vi "AnimatorCoordinator.vi"(8 "error in (no error)":errorcluster) -> (0 "error out":errorcluster)   [LabVIEW 2019, in "AnimatorXControl.xctl"]
uses:
  AnimatorXControl.xctl
  AnimatorSettings.ctl
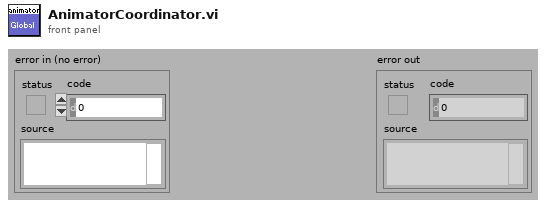
[diagram p1: front panel]
types:
  T1 = typedef "AnimatorXControl.xctl/AnimatorSettings.ctl" = cluster{"Reverse":bool, "FrameRate":dbl, "WorkMode":enum16{"Automatic", "UseValue"}}
  T2 = cluster{"Frame Interval":dbl, "Current Index":u32, "Left Interval":dbl, "Settings":T1}[]
  T3 = cluster{"Picture Ref":refnum<vi>, "PictureArray":picture[]}[]
  T4 = typedef "AnimatorXControl.xctl/QueueElement.ctl" = cluster{"Settings":T1, "Command":T5, "ImageInfo":cluster{"ImageData":picture[], "Pict Refnum":refnum<vi>}, "XRefnum":refnum<vi>}
  T5 = typedef "AnimatorXControl.xctl/AnimatorCommand.ctl" = enum16{"AddAnimator", "RemoveAnimator", "Settings"}
  T6 = cluster{"Frame Interval":dbl, "Current Index":u32, "Left Interval":dbl, "Settings":T1}
  T7 = cluster{"Picture Ref":refnum<vi>, "PictureArray":picture[]}
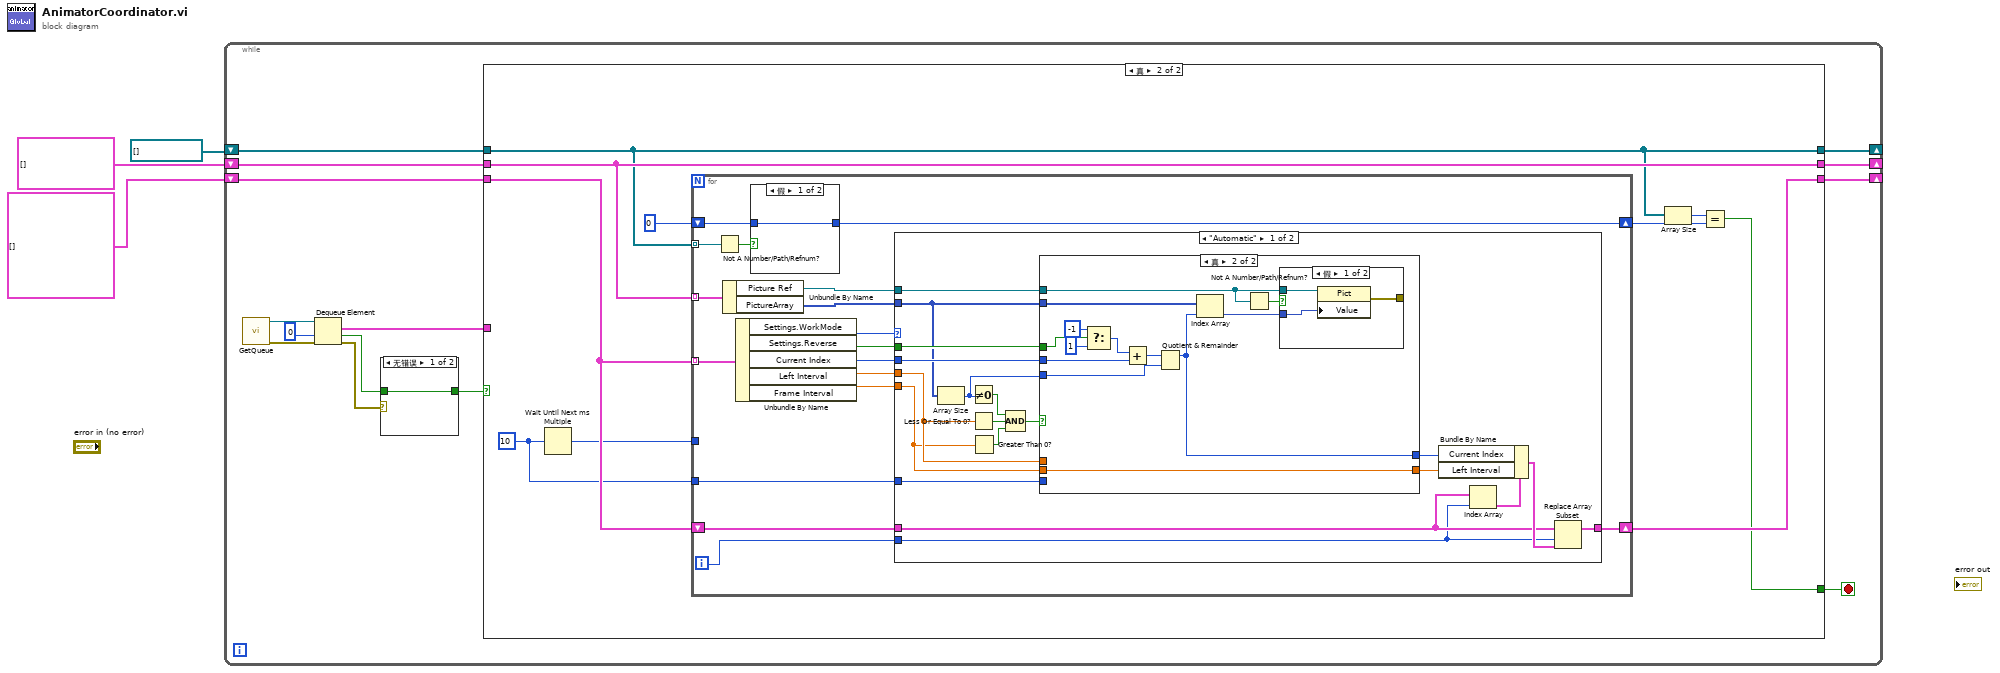
[diagram p0: block diagram]
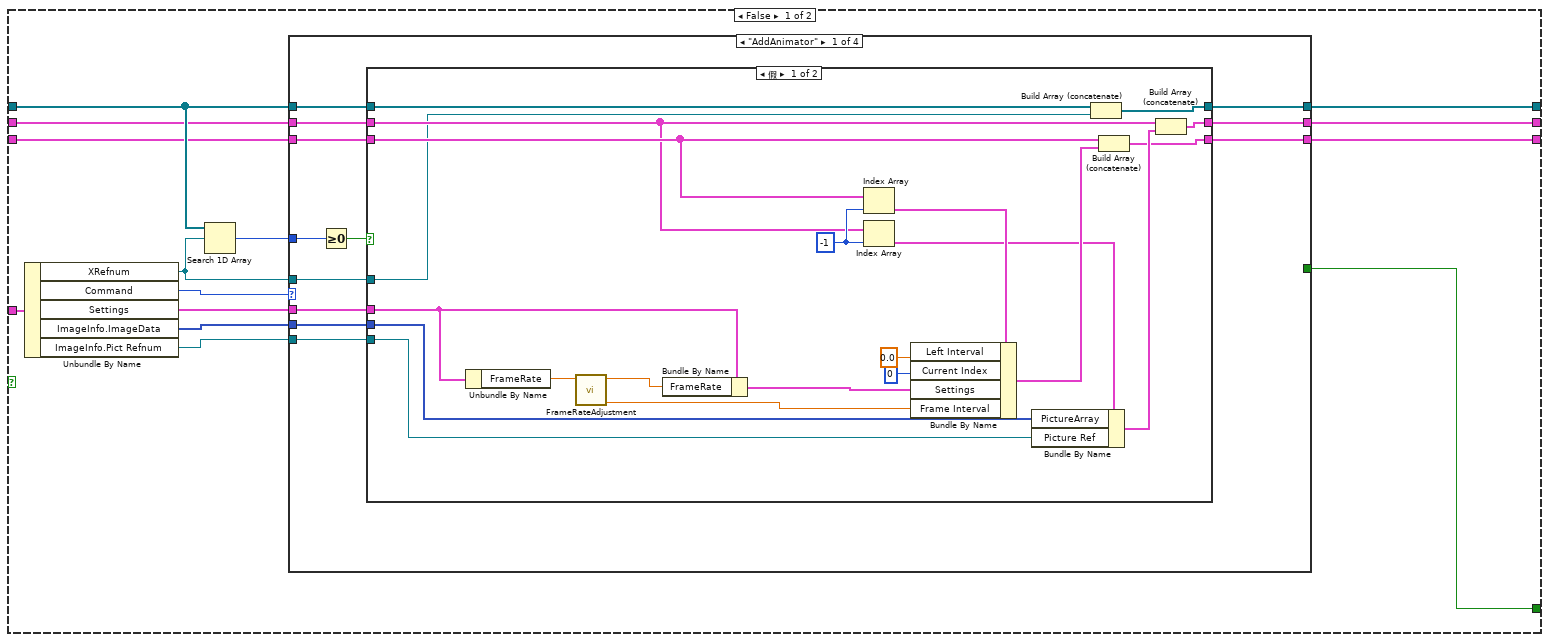
[diagram p2: hidden frame]
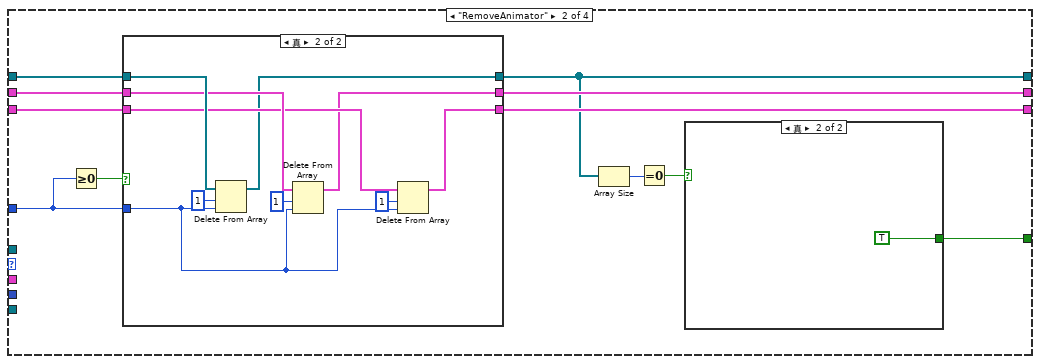
[diagram p4: hidden frame]
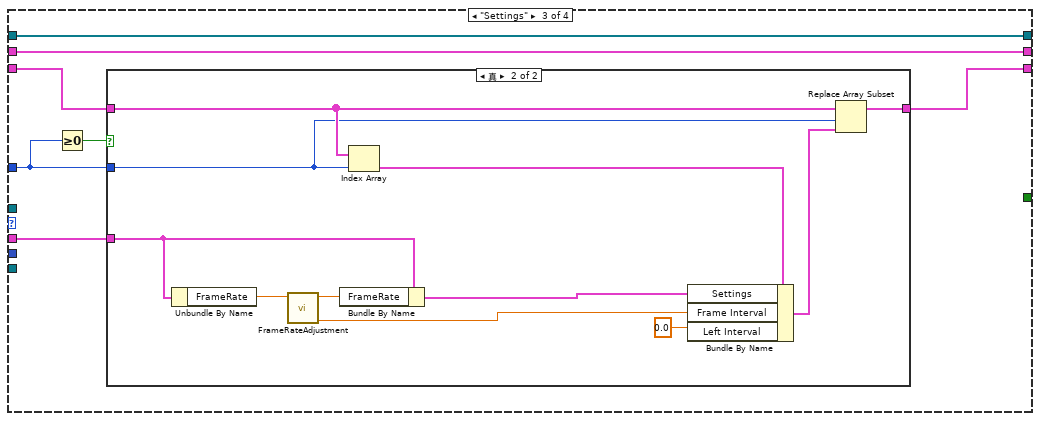
[diagram p7: hidden frame]
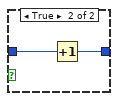
[diagram p10: hidden frame]
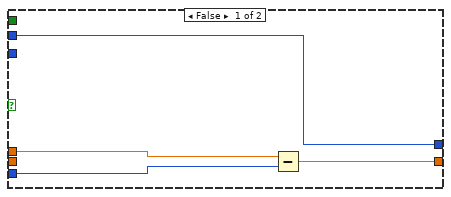
[diagram p11: hidden frame]
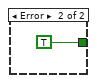
[diagram p14: hidden frame]
diagram:
  n1 = while {
    shift-right: [w15] -> _
    shift-left: refnum<vi>[] [] ("XControlRef Out") -> [w17]
    shift-right: [w13] -> _
    shift-left: T2 [] ("Settings Out") -> [w16]
    shift-right: [w11] -> _
    shift-left: T3 [] ("ImageData Out") -> [w12]
    stop <- w14 stop-if-true
    n2 = call "GetQueue.vi"() -> ("error out"=w8:errorcluster, "queue out"=w10:refnum<queue>)  [unwired: 10 in]
    n3 = Dequeue Element(queue=w10, timeout in ms (-1)=0, error in (no error)=w8) -> (element=w4:T4, timed out?=w6:bool, error out=w7:errorcluster)  [unwired: 1 out]
    n4 = case shown="无错误" w7 {
      tunnel: w6 -> [w185 _]
      tunnel: [w185 TRUE ("timed out?")] -> w5
      frame No Error {
      }
      frame Error {
      }
    }
    n5 = case shown="真" w5 {
      tunnel: w17 -> [w30 w118]
      tunnel: w16 -> [w28 w124]
      tunnel: [w27 w118] -> w15
      tunnel: [w18 w115] -> w14
      tunnel: [w25 w122] -> w13
      tunnel: w12 -> [w29 w123]
      tunnel: [w26 w123] -> w11
      tunnel: w4 -> [w31 _]
      frame False {
        n6 = Unbundle By Name(w31) -> ("XRefnum"=w23:refnum<vi>, "Command"=w24:T5, "Settings"=w20:T1, "ImageInfo.ImageData"=w19:picture[], "ImageInfo.Pict Refnum"=w22:refnum<vi>)
        n7 = Search 1D Array(1D array=w30, element=w23) -> (index of element=w21:i32)  [unwired: 1 in]
        n8 = case shown="\"AddAnimator\"" w24 {
          tunnel: w30 -> [w40 w78 w99 w114]
          tunnel: [w39 w71 w99 w114] -> w27
          tunnel: w29 -> [w41 w77 w97 w113]
          tunnel: w21 -> [w33 w73 w94 _]
          tunnel: [w38 w75 w97 w113] -> w26
          tunnel: w22 -> [w34 _ _ _]
          tunnel: w20 -> [w36 _ w98 _]
          tunnel: w19 -> [w35 _ _ _]
          tunnel: w28 -> [w42 w76 w96 w112]
          tunnel: [w43 w74 w95 w112] -> w25
          tunnel: w23 -> [w37 _ _ _]
          tunnel: [_ w68 _ _] -> w18
          frame "AddAnimator" {
            n9 = Greater Or Equal To 0?(x=w33) -> (x >= 0?=w32:bool)
            n10 = case shown="假" w32 {
              tunnel: [w58 w65] -> w43
              tunnel: w42 -> [w57 w65]
              tunnel: w41 -> [w56 w66]
              tunnel: w40 -> [w55 w67]
              tunnel: [w54 w67] -> w39
              tunnel: [w53 w66] -> w38
              tunnel: w37 -> [w52 _]
              tunnel: w36 -> [w48 _]
              tunnel: w35 -> [w51 _]
              tunnel: w34 -> [w50 _]
              frame False {
                w62 = -1
                n11 = Unbundle By Name(w48) -> ("FrameRate"=w49:dbl)
                n12 = call "FrameRateAdjustment.vi"("FrameRate In"=w49) -> ("FrameInterval"=w45:dbl, "FrameRate Out"=w47:dbl)  [unwired: 9 in]
                n13 = Bundle By Name(cluster=w48, "FrameRate"=w47) -> (w46:T1)
                n14 = Index Array(array=w57, index=w62) -> (element=w61:T6)
                n15 = Index Array(array=w56, index=w62) -> (element=w60:T7)
                n16 = Bundle By Name(cluster=w61, "Left Interval"=0.0, "Current Index"=u32 0, "Settings"=w46, "Frame Interval"=w45) -> (w63:T6)
                n17 = Bundle By Name(cluster=w60, "PictureArray"=w51, "Picture Ref"=w50) -> (w64:T7)
                n18 = Build Array (concatenate)(w55, w52) -> (w54:refnum<vi>[])
                n19 = Build Array (concatenate)(w57, w63) -> (w58:T2)
                n20 = Build Array (concatenate)(w56, w64) -> (w53:T3)
              }
              frame True {
              }
            }
          }
          frame "RemoveAnimator" {
            n21 = Greater Or Equal To 0?(x=w73) -> (x >= 0?=w72:bool)
            n22 = case shown="真" w72 {
              tunnel: w78 -> [w82 w89]
              tunnel: w77 -> [w81 w88]
              tunnel: w76 -> [w80 w87]
              tunnel: [w82 w83] -> w71
              tunnel: [w81 w86] -> w75
              tunnel: [w80 w85] -> w74
              tunnel: w73 -> [_ w84]
              frame False {
              }
              frame True {
                n23 = Delete From Array(array=w89, length=1, index=w84) -> (array with subset deleted=w83:refnum<vi>[])  [unwired: 1 out]
                n24 = Delete From Array(array=w88, length=1, index=w84) -> (array with subset deleted=w86:T3)  [unwired: 1 out]
                n25 = Delete From Array(array=w87, length=1, index=w84) -> (array with subset deleted=w85:T2)  [unwired: 1 out]
              }
            }
            n26 = Array Size(array=w71) -> (size(s)=w70:i32)
            n27 = Equal To 0?(x=w70) -> (x = 0?=w69:bool)
            n28 = case shown="真" w69 {
              tunnel: [_ TRUE] -> w68
              frame False {
              }
              frame True {
              }
            }
          }
          frame "Settings" {
            n29 = Greater Or Equal To 0?(x=w94) -> (x >= 0?=w93:bool)
            n30 = case shown="真" w93 {
              tunnel: w98 -> [_ w105]
              tunnel: w96 -> [w100 w110]
              tunnel: [w100 w109] -> w95
              tunnel: w94 -> [_ w107]
              frame False {
              }
              frame True {
                n31 = Unbundle By Name(w105) -> ("FrameRate"=w106:dbl)
                n32 = call "FrameRateAdjustment.vi"("FrameRate In"=w106) -> ("FrameInterval"=w103:dbl, "FrameRate Out"=w104:dbl)  [unwired: 9 in]
                n33 = Bundle By Name(cluster=w105, "FrameRate"=w104) -> (w102:T1)
                n34 = Index Array(array=w110, index=w107) -> (element=w111:T6)
                n35 = Bundle By Name(cluster=w111, "Settings"=w102, "Frame Interval"=w103, "Left Interval"=0.0) -> (w108:T6)
                n36 = Replace Array Subset(array=w110, new element=w108, index=w107) -> (w109:T2)
              }
            }
          }
          frame Default {
          }
        }
      }
      frame True {
        w120 = u32 10 ("millisecond multiple")
        n37 = Wait Until Next ms Multiple(millisecond multiple=w120) -> (millisecond timer value=w121:u32)
        n38 = for {
          tunnel: w120 -> [w136]
          shift-right: [w134] -> w122
          shift-left: w124 -> [w135]
          tunnel: w124 -> [w130] mode=indexing
          tunnel: w123 -> [w129] mode=indexing
          tunnel: w118 -> [w128] mode=indexing
          tunnel: w121 -> [_]
          shift-right: [w125] -> w117
          shift-left: u32 0 -> [w126]
          i -> [w131]
          n39 = Not A Number/Path/Refnum?(number/path/refnum=w128) -> (NaN/Path/Refnum?=w127:bool)
          n40 = Unbundle By Name(w129) -> ("Picture Ref"=w133:refnum<vi>, "PictureArray"=w132:picture[])
          n41 = Unbundle By Name(w130) -> ("Settings.WorkMode"=w141:enum16{"Automatic", "UseValue"}, "Settings.Reverse"=w138:bool, "Current Index"=w137:u32, "Left Interval"=w140:dbl, "Frame Interval"=w139:dbl)
          n42 = case shown="假" w127 {
            tunnel: w126 -> [w142 w144]
            tunnel: [w142 w143] -> w125
            frame False {
            }
            frame True {
              n43 = Increment(x=w144) -> (x+1=w143:u32)
            }
          }
          n44 = case shown="\"Automatic\"" w141 {
            tunnel: w133 -> [w156 _]
            tunnel: w140 -> [w155 _]
            tunnel: w139 -> [w154 _]
            tunnel: w137 -> [w158 _]
            tunnel: w138 -> [w159 _]
            tunnel: w136 -> [w153 _]
            tunnel: w135 -> [w148 w184]
            tunnel: w131 -> [w147 _]
            tunnel: [w146 w184] -> w134
            tunnel: w132 -> [w145 _]
            frame "Automatic" {
              n45 = Array Size(array=w145) -> (size(s)=w157:i32)
              n46 = Not Equal To 0?(x=w157) -> (x != 0?=w163:bool)
              n47 = Less Or Equal To 0?(x=w155) -> (x <= 0?=w162:bool)
              n48 = Greater Than 0?(x=w154) -> (x > 0?=w161:bool)
              n49 = Compound Arithmetic op=AND(w163, w162, w161) -> (w160:bool)
              n50 = case shown="真" w160 {
                tunnel: w159 -> [_ w178]
                tunnel: w158 -> [w164 w176]
                tunnel: w157 -> [_ w175]
                tunnel: w156 -> [_ w171]
                tunnel: w155 -> [w167 _]
                tunnel: w154 -> [_ w169]
                tunnel: w153 -> [w166 _]
                tunnel: [w165 w169] -> w150
                tunnel: [w164 w173] -> w151
                tunnel: w145 -> [_ w172]
                frame False {
                  n51 = Subtract(x=w167, y=w166) -> (x-y=w165:dbl)
                }
                frame True {
                  n52 = Select(t=-1, s=w178, f=1) -> (s? t:f=w177:i32)
                  n53 = Add(x=w177, y=w176) -> (x+y=w168:u32)
                  n54 = Quotient & Remainder(x=w168, y=w175) -> (x-y*floor(x/y)=w173:u32)  [unwired: 1 out]
                  n55 = Index Array(array=w172, index=w173) -> (element=w174:picture)
                  n56 = Not A Number/Path/Refnum?(number/path/refnum=w171) -> (NaN/Path/Refnum?=w170:bool)
                  n57 = case shown="假" w170 {
                    tunnel: w174 -> [w183 _]
                    tunnel: w171 -> [w182 _]
                    tunnel: [w181 _] -> _
                    frame False {
                      n58 = property class="Pict"(reference=w182, "Value"=w183) -> (error out=w181:errorcluster)  [unwired: 1 in, 1 out]
                    }
                    frame True {
                    }
                  }
                }
              }
              n59 = Index Array(array=w148, index=w147) -> (element=w152:T6)
              n60 = Bundle By Name(cluster=w152, "Current Index"=w151, "Left Interval"=w150) -> (w149:T6)
              n61 = Replace Array Subset(array=w148, new element=w149, index=w147) -> (w146:T2)
            }
            frame "UseValue", Default {
            }
          }
        }
        n62 = Array Size(array=w118) -> (size(s)=w116:i32)
        n63 = Equal?(x=w116, y=w117) -> (x = y?=w115:bool)
      }
    }
  }
